vi "题目6.vi"   [LabVIEW 2017]
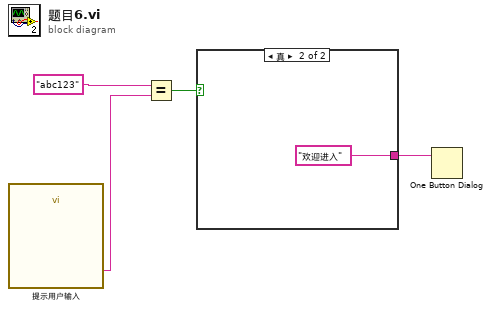
[diagram p0: block diagram]
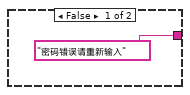
[diagram p2: hidden frame]
diagram:
  n1 = call "提示用户输入"() -> ("请输入密码"=w1:string)  [unwired: 16 in, 3 out]
  n2 = Equal?(x="abc123", y=w1) -> (x = y?=w2:bool)
  n3 = case shown="真" w2 {
    tunnel: ["密码错误请重新输入" "欢迎进入"] -> w4
    frame False {
    }
    frame True {
    }
  }
  n4 = One Button Dialog(message=w4) -> ()  [unwired: 1 in, 1 out]
